vi "Build Internal State String.vi"(5 "State":string, 7 "Arguments (\"\")":string, 9 "Arg-State (\"\")":string, 11 "Source (\"\")":string) -> (6 "State with Arguments":string)   [LabVIEW 2014, in "JKI State Machine++.lvlib"]
doc: "构建包含 JKI 状态机状态、参数等信息的字符串。\n\n<b>输入控件:</b>s\n - <b>State</b>: 状态字符串\n - <b>Arguments (\"\")</b>: <b>State</b>的参数\n - <b>Arg-State (\"\")</b>: 发送此消息的模块在发送此消息时处于的状态\n - <b>Source (\"\")</b>: 发送此消息的模块名称\n\n<b>输出控件:</b>\n - <b>State with Arguments</b>: 包含 JKI 状态机状态、参数等信息的字符串"
uses:
  JKI State Machine++.lvlib
panel:
  # "For instructions on how to use the JKI State Machine, examples and video tutorials, visit:\nhttp://jki.net/state-machine/\n\nJKI State Machine™\nhttp://jki.net/state-machine/\nCopyright (C) 2005-2017, JKI <info@jki.net>\nALL RIGHTS RESERVED"
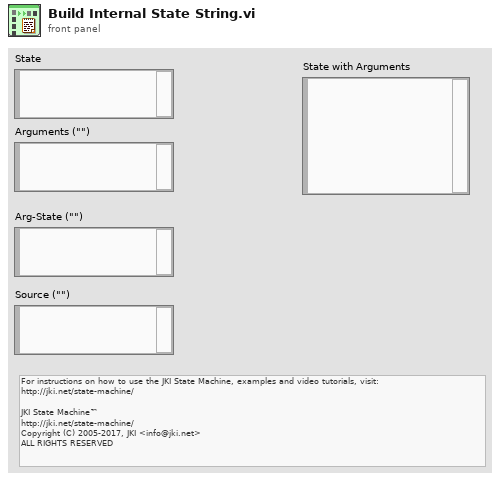
[diagram p1: front panel]
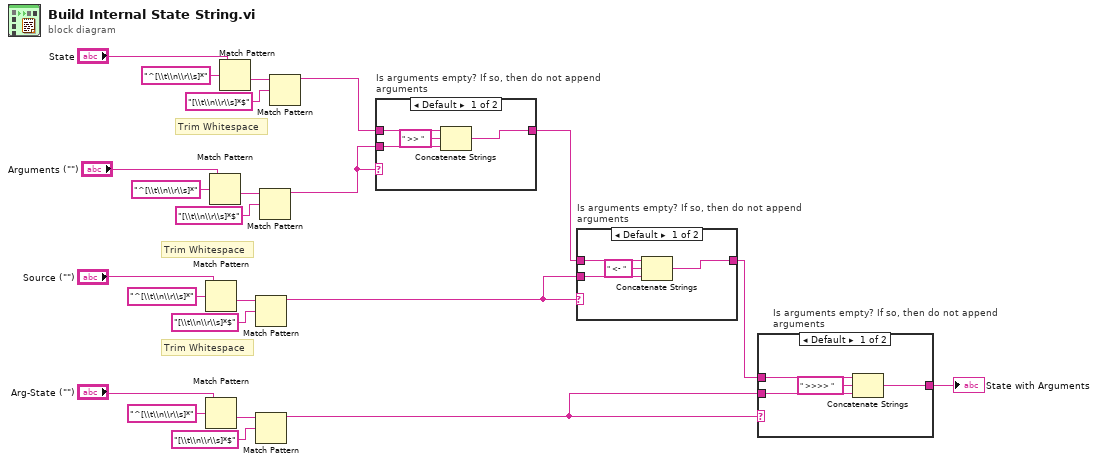
[diagram p0: block diagram]
diagram:
  # "Trim Whitespace"
  # "Trim Whitespace"
  # "Trim Whitespace"
  n1 = Match Pattern(string="Source (\"\")", regular expression="^[\\t\\n\\r\\s]*") -> (after substring=w12:string)  [unwired: 1 in, 3 out]
  n2 = Match Pattern(string="Arg-State (\"\")", regular expression="^[\\t\\n\\r\\s]*") -> (after substring=w7:string)  [unwired: 1 in, 3 out]
  n3 = Match Pattern(string="Arguments (\"\")", regular expression="^[\\t\\n\\r\\s]*") -> (after substring=w17:string)  [unwired: 1 in, 3 out]
  n4 = Match Pattern(string="State", regular expression="^[\\t\\n\\r\\s]*") -> (after substring=w22:string)  [unwired: 1 in, 3 out]
  n5 = Match Pattern(string=w12, regular expression="[\\t\\n\\r\\s]*$") -> (before substring=w9:string)  [unwired: 1 in, 3 out]
  n6 = Match Pattern(string=w7, regular expression="[\\t\\n\\r\\s]*$") -> (before substring=w4:string)  [unwired: 1 in, 3 out]
  n7 = Match Pattern(string=w17, regular expression="[\\t\\n\\r\\s]*$") -> (before substring=w14:string)  [unwired: 1 in, 3 out]
  n8 = Match Pattern(string=w22, regular expression="[\\t\\n\\r\\s]*$") -> (before substring=w19:string)  [unwired: 1 in, 3 out]
  n9 = case "Is arguments empty? If so, then do not append arguments" shown="Default" w14 {
    tunnel: [w24 w28] -> w3
    tunnel: w19 -> [w27 w28]
    tunnel: w14 -> [w25 _]
    frame Default {
      n10 = Concatenate Strings(w27, " >> " ("string"), w25) -> (w24:string)
    }
    frame "" {
    }
  }
  n11 = case "Is arguments empty? If so, then do not append arguments" shown="Default" w9 {
    tunnel: [w29 w33] -> w2
    tunnel: w3 -> [w32 w33]
    tunnel: w9 -> [w30 _]
    frame Default {
      n12 = Concatenate Strings(w32, " <- " ("string"), w30) -> (w29:string)
    }
    frame "" {
    }
  }
  n13 = case "Is arguments empty? If so, then do not append arguments" shown="Default" w4 {
    tunnel: [w35 w38] -> w1
    tunnel: w2 -> [w37 w38]
    tunnel: w4 -> [w36 _]
    frame Default {
      n14 = Concatenate Strings(w37, " >>>> " ("string"), w36) -> (w35:string)
    }
    frame "" {
    }
  }
  "State with Arguments" <- w1
